vi "The Final Demo.vi"   [LabVIEW 2016, in "Robot Project.lvrbt"]
uses:
  Robot Project.lvrbt
  <vilib>/NXT/Block Support/NXT_InputPort.ctl
  <vilib>/NXT/Block Support/NXT_OutputPort.ctl
  <vilib>/NXT/Dual Mode Library/Sensors/Touch_Pressed.vi
  <vilib>/NXT/Dual Mode Library/Sensors/EV3_Color_Color.vi
  <vilib>/NXT/NXTIO Xnodes/NXTIONodeSubVIs/NXTMoveMotors.vi
  <vilib>/NXT/Dual Mode Library/Waits/Wait_Num(msec).vi
  <vilib>/NXT/Dual Mode Library/Display/drawText.vi
  <vilib>/NXT/NXTIO Xnodes/NXTIONodeSubVIs/LEGOMotorStatus.vi
  <vilib>/NXT/Dual Mode Library/Display/drawNumber.vi
  <vilib>/NXT/Dual Mode Library/Waits/Wait_Num.vi
  <vilib>/NXT/NXTIO Xnodes/NXTIONodeSubVIs/NXTStopMotors.vi
  <vilib>/NXT/Subs/LVHSConnector.ctl
  <vilib>/NXT/NXTIO Xnodes/AddressXNode/NXTIOAddress.xnode
  test.lvrbt
  <vilib>/NXT/NXTIO Xnodes/NXTIOXNode/NXTIO.xnode
  <vilib>/NXT/LegoClasses/BrickReference/BrickReference.lvclass
types:
  T1 = typedef "NXT_InputPort.ctl" = u32
  T2 = typedef "LVHSConnector.ctl" = refnum<class "BrickReference.lvclass">
  T3 = typedef "ColorSensorColors.ctl" = enum16{"No Color", "Black", "Blue", "Green", "Yellow", "Red", "White", "Brown"}
  T4 = typedef "NXT_OutputPort.ctl" = u8
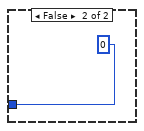
[diagram p8: hidden frame]
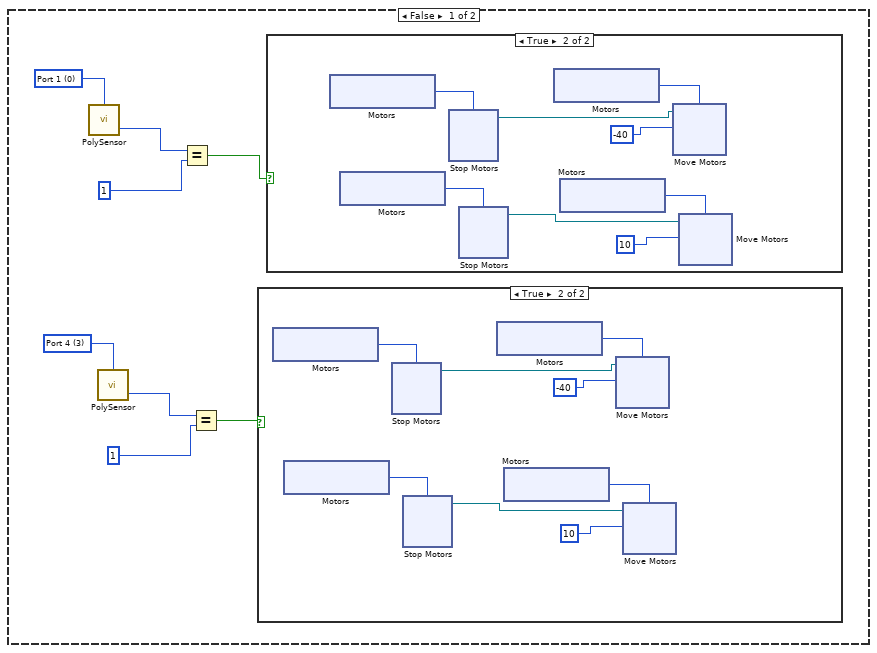
[diagram p10: hidden frame]
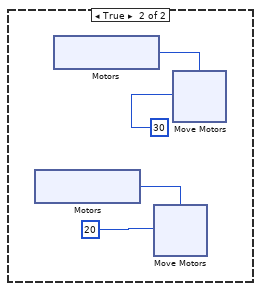
[diagram p17: hidden frame]
diagram:
  n1 = while {
    stop <- w1 continue-if-true
    n2 = while {
      shift-right: [w50] -> _
      shift-left: FALSE -> [w52]
      shift-right: [w41] -> _
      shift-left: 0 -> [w42]
      stop <- w54 continue-if-true
      w7 = T1 0 items=["Port 1", "Port 2", "Port 3", "Port 4"] ("Port (Port 1)")
      w10 = T1 3 items=["Port 1", "Port 2", "Port 3", "Port 4"] ("Port (Port 1)")
      w16 = T1 0 items=["Port 1", "Port 2", "Port 3", "Port 4"] ("Port (Port 1)")
      w19 = T1 3 items=["Port 1", "Port 2", "Port 3", "Port 4"] ("Port (Port 1)")
      w25 = T1 3 items=["Port 1", "Port 2", "Port 3", "Port 4"] ("Port (Port 1)")
      w31 = T1 0 items=["Port 1", "Port 2", "Port 3", "Port 4"] ("Port (Port 1)")
      w34 = T1 3 items=["Port 1", "Port 2", "Port 3", "Port 4"] ("Port (Port 1)")
      w37 = T1 0 items=["Port 1", "Port 2", "Port 3", "Port 4"] ("Port (Port 1)")
      w53 = T1 2 items=["Port 1", "Port 2", "Port 3", "Port 4"] ("Port (Port 1)")
      # "Left sensor"
      # "Right sensor"
      # "Left sensor"
      # "Right sensor"
      # "Right sensor"
      # "Left sensor"
      # "Right sensor"
      # "Left sensor"
      n3 = call-poly <vilib>:"PolySensor.vi"() -> ("Yes / No"=w54:bool)  [unwired: 3 in, 1 out]
      n4 = call-poly <vilib>:"PolySensor.vi"("Port (Port 1)"=w53) -> ("Yes / No"=w50:bool, "NXT/EV3"=w40:T2)  [unwired: 2 in]
      n5 = Not(x=w52) -> (.not. x?=w51:bool)
      n6 = And(x=w50, y=w51) -> (x .and. y?=w49:bool)
      n7 = call-poly <vilib>:"PolySensor.vi"("Port (Port 1)"=w10) -> ("Detected Color"=w11:T3)  [unwired: 2 in, 1 out]
      n8 = call-poly <vilib>:"PolySensor.vi"("Port (Port 1)"=w7) -> ("Detected Color"=w8:T3)  [unwired: 2 in, 1 out]
      n9 = Add(x=1, y=w42) -> (x+y=w47:i32)
      n10 = Select(t=w47, s=w49, f=w42) -> (s? t:f=w41:i32)
      n11 = Greater Or Equal?(x=w41, y=2) -> (x >= y?=w46:bool)
      n12 = Equal?(x=w41, y=1) -> (x = y?=w44:bool)
      n13 = case shown="True" w44 {
        tunnel: w40 -> [_ w185]
        frame False {
        }
        frame True {
          n14 = call-poly <vilib>:"PolyWait.vi"("Time (100 msec)"=20, "NXT/EV3"=w185) -> ("NXT/EV3"=w187:T2)  [unwired: 2 in]
          n15 = Wait (ms)(milliseconds to wait=2200) -> (millisecond timer value=w177:u32)
          n16 = xnode "Motors"() -> ("Motor"=w190:T4)
          n17 = xnode "Move Motors"("Power/Speed 1"=-20, "Motors"=w190, "NXT/EV3"=w187) -> ()  [unwired: 1 out]
          n18 = Greater Or Equal?(x=w177, y=2000) -> (x >= y?=w175:bool)
          n19 = xnode "Motors"() -> ("Motor"=w174:T4)
          n20 = xnode "Motors"() -> ("Motor"=w173:T4)
          n21 = xnode "Stop Motors"("Motors"=w174) -> ()  [unwired: 1 in, 1 out]
          n22 = xnode "Stop Motors"("Motors"=w173) -> ()  [unwired: 1 in, 1 out]
          n23 = case shown="True" w175 {
            tunnel: [w203 0] -> w169
            frame True {
              n24 = xnode "Motors"() -> ("Motor"=w206:T4)
              n25 = xnode "Motor Status"("Motors"=w206) -> ("Position 1"=w203:i32, "NXT/EV3"=w205:T2)  [unwired: 1 in, 1 out]
              n26 = call-poly <vilib>:"PolyDisplay.vi"("number"=w203, "NXT/EV3"=w205, "Line"=2) -> ()  [unwired: 1 in, 1 out]
            }
            frame False {
            }
          }
          n27 = Less Or Equal?(x=w169, y=340) -> (x <= y?=w171:bool)
          n28 = Greater?(x=w169, y=340) -> (0:w170:bool)
          n29 = Not Equal?(x=w169, y=0) -> (x != y?=w179:bool)
          n30 = And(x=w179, y=w171) -> (x .and. y?=w181:bool)
          n31 = case shown="True" w170 {
            frame False {
            }
            frame True {
              n32 = while {
                stop <- w235 continue-if-true
                w223 = T1 3 items=["Port 1", "Port 2", "Port 3", "Port 4"] ("Port (Port 1)")
                w226 = T1 0 items=["Port 1", "Port 2", "Port 3", "Port 4"] ("Port (Port 1)")
                w228 = T1 0 items=["Port 1", "Port 2", "Port 3", "Port 4"] ("Port (Port 1)")
                w234 = T1 3 items=["Port 1", "Port 2", "Port 3", "Port 4"] ("Port (Port 1)")
                # "drive code"
                n33 = call-poly <vilib>:"PolySensor.vi"("Port (Port 1)"=w226) -> ("Detected Color"=w225:T3)  [unwired: 2 in, 1 out]
                n34 = call-poly <vilib>:"PolySensor.vi"("Port (Port 1)"=w223) -> ("Detected Color"=w222:T3)  [unwired: 2 in, 1 out]
                n35 = Equal?(x=w225, y=6) -> (x = y?=w220:bool)
                n36 = Equal?(x=w222, y=6) -> (x = y?=w219:bool)
                n37 = And(x=w220, y=w219) -> (x .and. y?=w218:bool)
                n38 = case shown="True" w218 {
                  frame False {
                    w242 = T1 3 items=["Port 1", "Port 2", "Port 3", "Port 4"] ("Port (Port 1)")
                    w245 = T1 0 items=["Port 1", "Port 2", "Port 3", "Port 4"] ("Port (Port 1)")
                    n39 = call-poly <vilib>:"PolySensor.vi"("Port (Port 1)"=w245) -> ("Detected Color"=w244:T3)  [unwired: 2 in, 1 out]
                    n40 = call-poly <vilib>:"PolySensor.vi"("Port (Port 1)"=w242) -> ("Detected Color"=w241:T3)  [unwired: 2 in, 1 out]
                    n41 = Equal?(x=w244, y=1) -> (x = y?=w239:bool)
                    n42 = Equal?(x=w241, y=1) -> (x = y?=w238:bool)
                    n43 = case shown="True" w238 {
                      frame False {
                      }
                      frame True {
                        n44 = xnode "Motors"() -> ("Motor"=w253:T4)
                        n45 = xnode "Motors"() -> ("Motor"=w252:T4)
                        n46 = xnode "Stop Motors"("Motors"=w253) -> ("NXT/EV3"=w247:T2)  [unwired: 1 in]
                        n47 = xnode "Stop Motors"("Motors"=w252) -> ("NXT/EV3"=w246:T2)  [unwired: 1 in]
                        n48 = xnode "Motors"() -> ("Motor"=w251:T4)
                        n49 = xnode "Motors"() -> ("Motor"=w249:T4)
                        n50 = xnode "Move Motors"("Power/Speed 1"=-40, "Motors"=w251, "NXT/EV3"=w247) -> ()  [unwired: 1 out]
                        n51 = xnode "Move Motors"("Power/Speed 1"=10, "Motors"=w249, "NXT/EV3"=w246) -> ()  [unwired: 1 out]
                      }
                    }
                    n52 = case shown="True" w239 {
                      frame False {
                      }
                      frame True {
                        n53 = xnode "Motors"() -> ("Motor"=w289:T4)
                        n54 = xnode "Motors"() -> ("Motor"=w288:T4)
                        n55 = xnode "Stop Motors"("Motors"=w289) -> ("NXT/EV3"=w283:T2)  [unwired: 1 in]
                        n56 = xnode "Stop Motors"("Motors"=w288) -> ("NXT/EV3"=w282:T2)  [unwired: 1 in]
                        n57 = xnode "Motors"() -> ("Motor"=w287:T4)
                        n58 = xnode "Motors"() -> ("Motor"=w285:T4)
                        n59 = xnode "Move Motors"("Power/Speed 1"=-40, "Motors"=w287, "NXT/EV3"=w283) -> ()  [unwired: 1 out]
                        n60 = xnode "Move Motors"("Power/Speed 1"=10, "Motors"=w285, "NXT/EV3"=w282) -> ()  [unwired: 1 out]
                      }
                    }
                  }
                  frame True {
                    n61 = xnode "Motors"() -> ("Motor"=w320:T4)
                    n62 = xnode "Motors"() -> ("Motor"=w321:T4)
                    n63 = xnode "Move Motors"("Power/Speed 1"=20, "Motors"=w320) -> ()  [unwired: 1 in, 1 out]
                    n64 = xnode "Move Motors"("Power/Speed 1"=20, "Motors"=w321) -> ()  [unwired: 1 in, 1 out]
                  }
                }
                n65 = call-poly <vilib>:"PolySensor.vi"("Port (Port 1)"=w234) -> ("Detected Color"=w231:T3)  [unwired: 2 in, 1 out]
                n66 = call-poly <vilib>:"PolySensor.vi"("Port (Port 1)"=w228) -> ("Detected Color"=w227:T3)  [unwired: 2 in, 1 out]
                n67 = Equal?(x=w231, y=5) -> (x = y?=w233:bool)
                n68 = Equal?(x=w227, y=5) -> (x = y?=w232:bool)
                n69 = Or(x=w233, y=w232) -> (x .or. y?=w217:bool)
                n70 = case shown="True" w217 {
                  frame False {
                  }
                  frame True {
                    n71 = xnode "Motors"() -> ("Motor"=w399:T4)
                    n72 = xnode "Motors"() -> ("Motor"=w398:T4)
                    n73 = xnode "Motors"() -> ("Motor"=w373:T4)
                    n74 = xnode "Move Motors"("Power/Speed 1"=95, "Motors"=w399) -> ("NXT/EV3"=w390:T2)  [unwired: 1 in]
                    n75 = xnode "Move Motors"("Power/Speed 1"=-10, "Motors"=w398) -> ("NXT/EV3"=w387:T2)  [unwired: 1 in]
                    n76 = xnode "Motors"() -> ("Motor"=w381:T4)
                    n77 = xnode "Motors"() -> ("Motor"=w355:T4)
                    n78 = xnode "Motors"() -> ("Motor"=w356:T4)
                    n79 = call-poly <vilib>:"PolyWait.vi"("Time (1 sec)"=1, "NXT/EV3"=w387) -> ("NXT/EV3"=w386:T2)  [unwired: 2 in]
                    n80 = call-poly <vilib>:"PolyWait.vi"("Time (1 sec)"=1, "NXT/EV3"=w390) -> ("NXT/EV3"=w389:T2)  [unwired: 2 in]
                    n81 = xnode "Motors"() -> ("Motor"=w395:T4)
                    n82 = xnode "Motors"() -> ("Motor"=w394:T4)
                    n83 = xnode "Motors"() -> ("Motor"=w378:T4)
                    n84 = xnode "Motors"() -> ("Motor"=w376:T4)
                    n85 = xnode "Move Motors"("Power/Speed 1"=27, "Motors"=w395, "NXT/EV3"=w389) -> ("NXT/EV3"=w382:T2)
                    n86 = xnode "Move Motors"("Power/Speed 1"=25, "Motors"=w394, "NXT/EV3"=w386) -> ("NXT/EV3"=w383:T2)
                    n87 = call-poly <vilib>:"PolyWait.vi"("Time (1 sec)"=1, "NXT/EV3"=w382) -> ("NXT/EV3"=w346:T2)  [unwired: 2 in]
                    n88 = xnode "Motors"() -> ("Motor"=w345:T4)
                    n89 = xnode "Stop Motors"("Motors"=w345, "NXT/EV3"=w346) -> ("NXT/EV3"=w342:T2)
                    n90 = call-poly <vilib>:"PolyWait.vi"("Time (1 sec)"=1, "NXT/EV3"=w383) -> ("NXT/EV3"=w344:T2)  [unwired: 2 in]
                    n91 = call-poly <vilib>:"PolyWait.vi"("Time (1 sec)"=1, "NXT/EV3"=w342) -> ()  [unwired: 2 in, 1 out]
                    n92 = xnode "Motors"() -> ("Motor"=w343:T4)
                    n93 = xnode "Stop Motors"("Motors"=w343, "NXT/EV3"=w344) -> ("NXT/EV3"=w340:T2)
                    n94 = call-poly <vilib>:"PolyWait.vi"("Time (1 sec)"=1, "NXT/EV3"=w340) -> ("NXT/EV3"=w338:T2)  [unwired: 2 in]
                    n95 = xnode "Stop Motors"("Motors"=w373, "NXT/EV3"=w338) -> ("NXT/EV3"=w372:T2)
                    n96 = xnode "Move Motors"("Power/Speed 1"=-20, "Motors"=w381, "NXT/EV3"=w372) -> ("NXT/EV3"=w374:T2)
                    n97 = call-poly <vilib>:"PolyWait.vi"("Time (100 msec)"=2000, "NXT/EV3"=w374) -> ("NXT/EV3"=w371:T2)  [unwired: 2 in]
                    n98 = xnode "Move Motors"("Power/Speed 1"=-22, "Motors"=w378, "NXT/EV3"=w371) -> ("NXT/EV3"=w369:T2)
                    n99 = xnode "Move Motors"("Power/Speed 1"=-20, "Motors"=w376, "NXT/EV3"=w371) -> ("NXT/EV3"=w368:T2)
                    n100 = call-poly <vilib>:"PolyWait.vi"("Time (1 sec)"=1, "NXT/EV3"=w369) -> ("NXT/EV3"=w363:T2)  [unwired: 2 in]
                    n101 = call-poly <vilib>:"PolyWait.vi"("Time (1 sec)"=1, "NXT/EV3"=w368) -> ("NXT/EV3"=w361:T2)  [unwired: 2 in]
                    n102 = xnode "Motors"() -> ("Motor"=w366:T4)
                    n103 = xnode "Motors"() -> ("Motor"=w367:T4)
                    n104 = xnode "Move Motors"("Power/Speed 1"=18, "Motors"=w366, "NXT/EV3"=w361) -> ("NXT/EV3"=w357:T2)
                    n105 = xnode "Move Motors"("Power/Speed 1"=-95, "Motors"=w367, "NXT/EV3"=w363) -> ("NXT/EV3"=w358:T2)
                    n106 = call-poly <vilib>:"PolyWait.vi"("Time (1 sec)"=1, "NXT/EV3"=w358) -> ("NXT/EV3"=w351:T2)  [unwired: 2 in]
                    n107 = xnode "Move Motors"("Power/Speed 1"=25, "Motors"=w356, "NXT/EV3"=w351) -> ("NXT/EV3"=w348:T2)
                    n108 = call-poly <vilib>:"PolyWait.vi"("Time (1 sec)"=1.5, "NXT/EV3"=w348) -> ()  [unwired: 2 in, 1 out]
                    n109 = call-poly <vilib>:"PolyWait.vi"("Time (1 sec)"=1, "NXT/EV3"=w357) -> ("NXT/EV3"=w352:T2)  [unwired: 2 in]
                    n110 = xnode "Move Motors"("Power/Speed 1"=27, "Motors"=w355, "NXT/EV3"=w352) -> ("NXT/EV3"=w347:T2)
                    n111 = call-poly <vilib>:"PolyWait.vi"("Time (1 sec)"=1.5, "NXT/EV3"=w347) -> ()  [unwired: 2 in, 1 out]
                  }
                }
                n112 = call-poly <vilib>:"PolyDisplay.vi"("Text"="light", "Line"=4) -> ()  [unwired: 2 in, 1 out]
                n113 = call-poly <vilib>:"PolySensor.vi"() -> ("Yes / No"=w235:bool)  [unwired: 3 in, 1 out]
              }
            }
          }
          n114 = case shown="True" w181 {
            frame False {
            }
            frame True {
              n115 = while {
                stop <- w524 continue-if-true
                w511 = T1 3 items=["Port 1", "Port 2", "Port 3", "Port 4"] ("Port (Port 1)")
                w514 = T1 0 items=["Port 1", "Port 2", "Port 3", "Port 4"] ("Port (Port 1)")
                w522 = T1 0 items=["Port 1", "Port 2", "Port 3", "Port 4"] ("Port (Port 1)")
                w523 = T1 3 items=["Port 1", "Port 2", "Port 3", "Port 4"] ("Port (Port 1)")
                # "drive code"
                # "drive program"
                n116 = call-poly <vilib>:"PolySensor.vi"("Port (Port 1)"=w514) -> ("Detected Color"=w513:T3)  [unwired: 2 in, 1 out]
                n117 = call-poly <vilib>:"PolySensor.vi"("Port (Port 1)"=w511) -> ("Detected Color"=w510:T3)  [unwired: 2 in, 1 out]
                n118 = Equal?(x=w513, y=6) -> (x = y?=w508:bool)
                n119 = Equal?(x=w510, y=6) -> (x = y?=w507:bool)
                n120 = And(x=w508, y=w507) -> (x .and. y?=w506:bool)
                n121 = case shown="False" w506 {
                  frame False {
                    w533 = T1 3 items=["Port 1", "Port 2", "Port 3", "Port 4"] ("Port (Port 1)")
                    w536 = T1 0 items=["Port 1", "Port 2", "Port 3", "Port 4"] ("Port (Port 1)")
                    n122 = call-poly <vilib>:"PolySensor.vi"("Port (Port 1)"=w533) -> ("Detected Color"=w532:T3)  [unwired: 2 in, 1 out]
                    n123 = call-poly <vilib>:"PolySensor.vi"("Port (Port 1)"=w536) -> ("Detected Color"=w535:T3)  [unwired: 2 in, 1 out]
                    n124 = Equal?(x=w532, y=1) -> (x = y?=w529:bool)
                    n125 = Equal?(x=w535, y=1) -> (x = y?=w530:bool)
                    n126 = case shown="True" w529 {
                      frame False {
                      }
                      frame True {
                        n127 = xnode "Motors"() -> ("Motor"=w544:T4)
                        n128 = xnode "Motors"() -> ("Motor"=w543:T4)
                        n129 = xnode "Stop Motors"("Motors"=w544) -> ("NXT/EV3"=w538:T2)  [unwired: 1 in]
                        n130 = xnode "Stop Motors"("Motors"=w543) -> ("NXT/EV3"=w537:T2)  [unwired: 1 in]
                        n131 = xnode "Motors"() -> ("Motor"=w542:T4)
                        n132 = xnode "Motors"() -> ("Motor"=w540:T4)
                        n133 = xnode "Move Motors"("Power/Speed 1"=40, "Motors"=w542, "NXT/EV3"=w538) -> ()  [unwired: 1 out]
                        n134 = xnode "Move Motors"("Power/Speed 1"=10, "Motors"=w540, "NXT/EV3"=w537) -> ()  [unwired: 1 out]
                      }
                    }
                    n135 = case shown="True" w530 {
                      frame False {
                      }
                      frame True {
                        n136 = xnode "Motors"() -> ("Motor"=w580:T4)
                        n137 = xnode "Motors"() -> ("Motor"=w579:T4)
                        n138 = xnode "Stop Motors"("Motors"=w580) -> ("NXT/EV3"=w574:T2)  [unwired: 1 in]
                        n139 = xnode "Stop Motors"("Motors"=w579) -> ("NXT/EV3"=w573:T2)  [unwired: 1 in]
                        n140 = xnode "Motors"() -> ("Motor"=w578:T4)
                        n141 = xnode "Motors"() -> ("Motor"=w576:T4)
                        n142 = xnode "Move Motors"("Power/Speed 1"=40, "Motors"=w578, "NXT/EV3"=w574) -> ()  [unwired: 1 out]
                        n143 = xnode "Move Motors"("Power/Speed 1"=10, "Motors"=w576, "NXT/EV3"=w573) -> ()  [unwired: 1 out]
                      }
                    }
                  }
                  frame True {
                    n144 = xnode "Motors"() -> ("Motor"=w611:T4)
                    n145 = xnode "Motors"() -> ("Motor"=w612:T4)
                    n146 = xnode "Move Motors"("Power/Speed 1"=20, "Motors"=w611) -> ()  [unwired: 1 in, 1 out]
                    n147 = xnode "Move Motors"("Power/Speed 1"=30, "Motors"=w612) -> ()  [unwired: 1 in, 1 out]
                  }
                }
                n148 = call-poly <vilib>:"PolySensor.vi"("Port (Port 1)"=w523) -> ("Detected Color"=w519:T3)  [unwired: 2 in, 1 out]
                n149 = call-poly <vilib>:"PolySensor.vi"("Port (Port 1)"=w522) -> ("Detected Color"=w518:T3)  [unwired: 2 in, 1 out]
                n150 = call-poly <vilib>:"PolyDisplay.vi"("Text"="heavey", "Line"=4) -> ()  [unwired: 2 in, 1 out]
                n151 = Equal?(x=w519, y=3) -> (x = y?=w521:bool)
                n152 = Equal?(x=w518, y=3) -> (x = y?=w520:bool)
                n153 = xnode "Motors"() -> ("Motor"=w526:T4)
                n154 = Or(x=w521, y=w520) -> (x .or. y?=w515:bool)
                n155 = case shown="True" w515 {
                  frame False {
                  }
                  frame True {
                    w634 = T1 3 items=["Port 1", "Port 2", "Port 3", "Port 4"] ("Port (Port 1)")
                    w637 = T1 0 items=["Port 1", "Port 2", "Port 3", "Port 4"] ("Port (Port 1)")
                    n156 = xnode "Motors"() -> ("Motor"=w691:T4)
                    n157 = xnode "Motors"() -> ("Motor"=w690:T4)
                    n158 = xnode "Motors"() -> ("Motor"=w665:T4)
                    n159 = xnode "Move Motors"("Power/Speed 1"=95, "Motors"=w691) -> ("NXT/EV3"=w682:T2)  [unwired: 1 in]
                    n160 = xnode "Move Motors"("Power/Speed 1"=-10, "Motors"=w690) -> ("NXT/EV3"=w679:T2)  [unwired: 1 in]
                    n161 = xnode "Motors"() -> ("Motor"=w673:T4)
                    n162 = xnode "Motors"() -> ("Motor"=w646:T4)
                    n163 = xnode "Motors"() -> ("Motor"=w647:T4)
                    n164 = call-poly <vilib>:"PolyWait.vi"("Time (1 sec)"=1, "NXT/EV3"=w682) -> ("NXT/EV3"=w681:T2)  [unwired: 2 in]
                    n165 = call-poly <vilib>:"PolyWait.vi"("Time (1 sec)"=1, "NXT/EV3"=w679) -> ("NXT/EV3"=w678:T2)  [unwired: 2 in]
                    n166 = call-poly <vilib>:"PolySensor.vi"("Port (Port 1)"=w637) -> ("Detected Color"=w636:T3)  [unwired: 2 in, 1 out]
                    n167 = call-poly <vilib>:"PolySensor.vi"("Port (Port 1)"=w634) -> ("Detected Color"=w633:T3)  [unwired: 2 in, 1 out]
                    n168 = Equal?(x=w636, y=6) -> (x = y?=w631:bool)
                    n169 = xnode "Motors"() -> ("Motor"=w687:T4)
                    n170 = xnode "Motors"() -> ("Motor"=w686:T4)
                    n171 = Equal?(x=w633, y=6) -> (x = y?=w630:bool)
                    n172 = xnode "Motors"() -> ("Motor"=w670:T4)
                    n173 = xnode "Motors"() -> ("Motor"=w668:T4)
                    n174 = xnode "Move Motors"("Power/Speed 1"=27, "Motors"=w687, "NXT/EV3"=w681) -> ("NXT/EV3"=w674:T2)
                    n175 = xnode "Move Motors"("Power/Speed 1"=25, "Motors"=w686, "NXT/EV3"=w678) -> ("NXT/EV3"=w675:T2)
                    n176 = Or(x=w631, y=w630) -> (x .or. y?=w629:bool)
                    n177 = call-poly <vilib>:"PolyWait.vi"("Time (1 sec)"=1, "NXT/EV3"=w674) -> ()  [unwired: 2 in, 1 out]
                    n178 = case shown="True" w629 {
                      frame False {
                      }
                      frame True {
                        n179 = while {
                          stop <- w692 continue-if-true
                          w698 = T1 3 items=["Port 1", "Port 2", "Port 3", "Port 4"] ("Port (Port 1)")
                          w701 = T1 0 items=["Port 1", "Port 2", "Port 3", "Port 4"] ("Port (Port 1)")
                          n180 = call-poly <vilib>:"PolySensor.vi"("Port (Port 1)"=w701) -> ("Detected Color"=w700:T3)  [unwired: 2 in, 1 out]
                          n181 = call-poly <vilib>:"PolySensor.vi"("Port (Port 1)"=w698) -> ("Detected Color"=w697:T3)  [unwired: 2 in, 1 out]
                          n182 = Equal?(x=w700, y=6) -> (x = y?=w695:bool)
                          n183 = Equal?(x=w697, y=6) -> (x = y?=w694:bool)
                          n184 = And(x=w695, y=w694) -> (x .and. y?=w693:bool)
                          n185 = case shown="False" w693 {
                            frame False {
                              w706 = T1 3 items=["Port 1", "Port 2", "Port 3", "Port 4"] ("Port (Port 1)")
                              w709 = T1 0 items=["Port 1", "Port 2", "Port 3", "Port 4"] ("Port (Port 1)")
                              n186 = call-poly <vilib>:"PolySensor.vi"("Port (Port 1)"=w706) -> ("Detected Color"=w705:T3)  [unwired: 2 in, 1 out]
                              n187 = call-poly <vilib>:"PolySensor.vi"("Port (Port 1)"=w709) -> ("Detected Color"=w708:T3)  [unwired: 2 in, 1 out]
                              n188 = Equal?(x=w705, y=1) -> (x = y?=w702:bool)
                              n189 = Equal?(x=w708, y=1) -> (x = y?=w703:bool)
                              n190 = case shown="True" w702 {
                                frame False {
                                }
                                frame True {
                                n191 = xnode "Motors"() -> ("Motor"=w717:T4)
                                n192 = xnode "Motors"() -> ("Motor"=w716:T4)
                                n193 = xnode "Stop Motors"("Motors"=w717) -> ("NXT/EV3"=w711:T2)  [unwired: 1 in]
                                n194 = xnode "Stop Motors"("Motors"=w716) -> ("NXT/EV3"=w710:T2)  [unwired: 1 in]
                                n195 = xnode "Motors"() -> ("Motor"=w715:T4)
                                n196 = xnode "Motors"() -> ("Motor"=w713:T4)
                                n197 = xnode "Move Motors"("Power/Speed 1"=40, "Motors"=w715, "NXT/EV3"=w711) -> ()  [unwired: 1 out]
                                n198 = xnode "Move Motors"("Power/Speed 1"=-10, "Motors"=w713, "NXT/EV3"=w710) -> ()  [unwired: 1 out]
                                }
                              }
                              n199 = case shown="True" w703 {
                                frame False {
                                }
                                frame True {
                                n200 = xnode "Motors"() -> ("Motor"=w753:T4)
                                n201 = xnode "Motors"() -> ("Motor"=w752:T4)
                                n202 = xnode "Stop Motors"("Motors"=w753) -> ("NXT/EV3"=w747:T2)  [unwired: 1 in]
                                n203 = xnode "Stop Motors"("Motors"=w752) -> ("NXT/EV3"=w746:T2)  [unwired: 1 in]
                                n204 = xnode "Motors"() -> ("Motor"=w751:T4)
                                n205 = xnode "Motors"() -> ("Motor"=w749:T4)
                                n206 = xnode "Move Motors"("Power/Speed 1"=40, "Motors"=w751, "NXT/EV3"=w747) -> ()  [unwired: 1 out]
                                n207 = xnode "Move Motors"("Power/Speed 1"=-10, "Motors"=w749, "NXT/EV3"=w746) -> ()  [unwired: 1 out]
                                }
                              }
                            }
                            frame True {
                              n208 = xnode "Motors"() -> ("Motor"=w784:T4)
                              n209 = xnode "Motors"() -> ("Motor"=w785:T4)
                              n210 = xnode "Move Motors"("Power/Speed 1"=-20, "Motors"=w784) -> ()  [unwired: 1 in, 1 out]
                              n211 = xnode "Move Motors"("Power/Speed 1"=-30, "Motors"=w785) -> ()  [unwired: 1 in, 1 out]
                            }
                          }
                          n212 = call-poly <vilib>:"PolySensor.vi"() -> ("Yes / No"=w692:bool)  [unwired: 3 in, 1 out]
                        }
                      }
                    }
                    n213 = call-poly <vilib>:"PolyWait.vi"("Time (1 sec)"=1, "NXT/EV3"=w675) -> ("NXT/EV3"=w662:T2)  [unwired: 2 in]
                    n214 = xnode "Stop Motors"("Motors"=w665, "NXT/EV3"=w662) -> ("NXT/EV3"=w664:T2)
                    n215 = xnode "Move Motors"("Power/Speed 1"=20, "Motors"=w673, "NXT/EV3"=w664) -> ("NXT/EV3"=w666:T2)
                    n216 = call-poly <vilib>:"PolyWait.vi"("Time (100 msec)"=2000, "NXT/EV3"=w666) -> ("NXT/EV3"=w663:T2)  [unwired: 2 in]
                    n217 = xnode "Move Motors"("Power/Speed 1"=-15, "Motors"=w670, "NXT/EV3"=w663) -> ("NXT/EV3"=w660:T2)
                    n218 = xnode "Move Motors"("Power/Speed 1"=15, "Motors"=w668, "NXT/EV3"=w663) -> ("NXT/EV3"=w659:T2)
                    n219 = call-poly <vilib>:"PolyWait.vi"("Time (1 sec)"=0.6, "NXT/EV3"=w660) -> ("NXT/EV3"=w654:T2)  [unwired: 2 in]
                    n220 = call-poly <vilib>:"PolyWait.vi"("Time (1 sec)"=1.3, "NXT/EV3"=w659) -> ("NXT/EV3"=w652:T2)  [unwired: 2 in]
                    n221 = xnode "Motors"() -> ("Motor"=w657:T4)
                    n222 = xnode "Motors"() -> ("Motor"=w658:T4)
                    n223 = xnode "Move Motors"("Power/Speed 1"=18, "Motors"=w657, "NXT/EV3"=w652) -> ("NXT/EV3"=w648:T2)
                    n224 = xnode "Move Motors"("Power/Speed 1"=-95, "Motors"=w658, "NXT/EV3"=w654) -> ("NXT/EV3"=w649:T2)
                    n225 = call-poly <vilib>:"PolyWait.vi"("Time (1 sec)"=1.1, "NXT/EV3"=w649) -> ("NXT/EV3"=w642:T2)  [unwired: 2 in]
                    n226 = xnode "Move Motors"("Power/Speed 1"=25, "Motors"=w647, "NXT/EV3"=w642) -> ("NXT/EV3"=w639:T2)
                    n227 = call-poly <vilib>:"PolyWait.vi"("Time (1 sec)"=1, "NXT/EV3"=w639) -> ()  [unwired: 2 in, 1 out]
                    n228 = call-poly <vilib>:"PolyWait.vi"("Time (1 sec)"=1.1, "NXT/EV3"=w648) -> ("NXT/EV3"=w643:T2)  [unwired: 2 in]
                    n229 = xnode "Move Motors"("Power/Speed 1"=27, "Motors"=w646, "NXT/EV3"=w643) -> ("NXT/EV3"=w638:T2)
                    n230 = call-poly <vilib>:"PolyWait.vi"("Time (1 sec)"=1, "NXT/EV3"=w638) -> ()  [unwired: 2 in, 1 out]
                  }
                }
                n231 = xnode "Move Motors"("Power/Speed 1"=90, "Motors"=w526) -> ()  [unwired: 1 in, 1 out]
                n232 = call-poly <vilib>:"PolySensor.vi"() -> ("Yes / No"=w524:bool)  [unwired: 3 in, 1 out]
              }
            }
          }
          n233 = call-poly <vilib>:"PolyDisplay.vi"("Text"="motor rotations", "Line"=1) -> ()  [unwired: 2 in, 1 out]
          n234 = call-poly <vilib>:"PolyDisplay.vi"("Text"="class", "Line"=3) -> ()  [unwired: 2 in, 1 out]
        }
      }
      n235 = case shown="True" w46 {
        frame False {
        }
        frame True {
          n236 = xnode "Motors"() -> ("Motor"=w143:T4)
          n237 = xnode "Move Motors"("Power/Speed 1"=-20, "Motors"=w143) -> ("NXT/EV3"=w136:T2)  [unwired: 1 in]
          n238 = call-poly <vilib>:"PolyWait.vi"("Time (100 msec)"=2000, "NXT/EV3"=w136) -> ("NXT/EV3"=w135:T2)  [unwired: 2 in]
          n239 = xnode "Motors"() -> ("Motor"=w140:T4)
          n240 = xnode "Motors"() -> ("Motor"=w138:T4)
          n241 = xnode "Move Motors"("Power/Speed 1"=-20, "Motors"=w140, "NXT/EV3"=w135) -> ()  [unwired: 1 out]
          n242 = xnode "Move Motors"("Power/Speed 1"=-20, "Motors"=w138, "NXT/EV3"=w135) -> ()  [unwired: 1 out]
        }
      }
      n243 = Equal?(x=w8, y=6) -> (x = y?=w6:bool)
      n244 = call-poly <vilib>:"PolySensor.vi"("Port (Port 1)"=w16) -> ("Detected Color"=w17:T3)  [unwired: 2 in, 1 out]
      n245 = call-poly <vilib>:"PolySensor.vi"("Port (Port 1)"=w37) -> ("Detected Color"=w38:T3)  [unwired: 2 in, 1 out]
      n246 = call-poly <vilib>:"PolySensor.vi"("Port (Port 1)"=w25) -> ("Detected Color"=w26:T3)  [unwired: 2 in, 1 out]
      n247 = call-poly <vilib>:"PolySensor.vi"("Port (Port 1)"=w34) -> ("Detected Color"=w35:T3)  [unwired: 2 in, 1 out]
      n248 = call-poly <vilib>:"PolySensor.vi"("Port (Port 1)"=w31) -> ("Detected Color"=w32:T3)  [unwired: 2 in, 1 out]
      n249 = call-poly <vilib>:"PolySensor.vi"("Port (Port 1)"=w19) -> ("Detected Color"=w20:T3)  [unwired: 2 in, 1 out]
      n250 = Equal?(x=w11, y=6) -> (x = y?=w5:bool)
      n251 = Equal?(x=w38, y=1) -> (x = y?=w23:bool)
      n252 = Equal?(x=w32, y=6) -> (x = y?=w29:bool)
      n253 = Equal?(x=w17, y=1) -> (x = y?=w14:bool)
      n254 = And(x=w5, y=w6) -> (x .and. y?=w4:bool)
      n255 = Equal?(x=w26, y=6) -> (x = y?=w24:bool)
      n256 = Equal?(x=w35, y=1) -> (x = y?=w28:bool)
      n257 = Equal?(x=w20, y=1) -> (x = y?=w13:bool)
      n258 = And(x=w23, y=w24) -> (x .and. y?=w22:bool)
      n259 = And(x=w28, y=w29) -> (x .and. y?=w30:bool)
      n260 = And(x=w13, y=w14) -> (x .and. y?=w15:bool)
      n261 = case shown="True" w4 {
        frame False {
        }
        frame True {
          # "Connected to left motor"
          # "Connected to right motor"
          # "Go straight"
          n262 = xnode "Motors"() -> ("Motor"=w56:T4)
          n263 = xnode "Motors"() -> ("Motor"=w58:T4)
          n264 = xnode "Move Motors"("Power/Speed 1"=15, "Motors"=w58) -> ()  [unwired: 1 in, 1 out]
          n265 = xnode "Move Motors"("Power/Speed 1"=15, "Motors"=w56) -> ()  [unwired: 1 in, 1 out]
        }
      }
      n266 = case shown="True" w22 {
        frame False {
        }
        frame True {
          # "Connected to left motor"
          # "connected to right motor"
          # "Turn Left"
          n267 = xnode "Motors"() -> ("Motor"=w117:T4)
          n268 = xnode "Motors"() -> ("Motor"=w118:T4)
          n269 = xnode "Move Motors"("Power/Speed 1"=-8, "Motors"=w118) -> ()  [unwired: 1 in, 1 out]
          n270 = xnode "Move Motors"("Power/Speed 1"=95, "Motors"=w117) -> ()  [unwired: 1 in, 1 out]
        }
      }
      n271 = case shown="True" w30 {
        frame False {
        }
        frame True {
          # "Connected to left motor"
          # "Connected to right motor"
          # "Turn Right"
          n272 = xnode "Motors"() -> ("Motor"=w96:T4)
          n273 = xnode "Motors"() -> ("Motor"=w98:T4)
          n274 = xnode "Move Motors"("Power/Speed 1"=-8, "Motors"=w96) -> ()  [unwired: 1 in, 1 out]
          n275 = xnode "Move Motors"("Power/Speed 1"=95, "Motors"=w98) -> ()  [unwired: 1 in, 1 out]
        }
      }
      n276 = case shown="True" w15 {
        frame False {
        }
        frame True {
          # "Connected to left motor"
          # "Connected to right motor"
          # "Go straight"
          n277 = xnode "Motors"() -> ("Motor"=w77:T4)
          n278 = xnode "Motors"() -> ("Motor"=w78:T4)
          n279 = xnode "Move Motors"("Power/Speed 1"=15, "Motors"=w78) -> ()  [unwired: 1 in, 1 out]
          n280 = xnode "Move Motors"("Power/Speed 1"=15, "Motors"=w77) -> ()  [unwired: 1 in, 1 out]
        }
      }
    }
    n281 = call-poly <vilib>:"PolySensor.vi"() -> ("Yes / No"=w1:bool)  [unwired: 3 in, 1 out]
  }
